vi "Get Model Data.vi"(8 "error in (no error)":errorcluster, 11 "Result Model by Reference In":refnum<class "Result Model by Reference.lvclass">) -> (0 "error out":errorcluster, 2 "Model Data":refnum<class "Result Model.lvclass">)   [LabVIEW 2020, in "Result Model by Reference.lvclass"]
uses:
  Result Model by Reference.lvclass
  Result Model by Reference.lvclass/Result Model by Reference.ctl
  Result Model/Result Model.lvclass
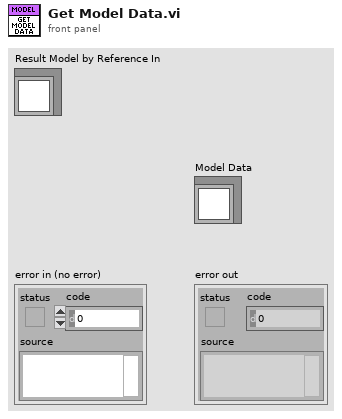
[diagram p1: front panel]
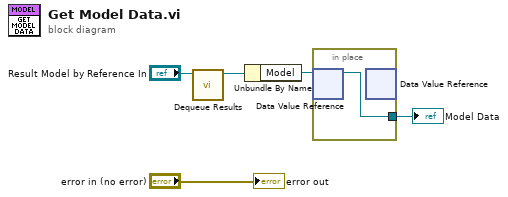
[diagram p0: block diagram]
diagram:
  n1 = call "Dequeue Results.vi"("Result Model by Reference in"="Result Model by Reference In") -> ("Result Model by Reference out"=w1:refnum<class "Result Model by Reference.lvclass">)  [unwired: 10 in]
  n2 = Unbundle By Name(w1) -> ("Model"=w5:refnum<data-value>)
  n3 = in-place {
    in-place-border: [w6] -> w4
    n4 = in-place-dvr #1(w5) -> (w6:refnum<class "Result Model.lvclass">)  [unwired: 1 out]
    n5 = in-place-dvr #1() -> ()  [unwired: 1 in, 2 out]
  }
  "Model Data" <- w4
  "error out" <- "error in (no error)"
